vi "Initialize Ramp.vi"(7 "Sample Count":dbl, 8 "error in (no error)":errorcluster, 9 "End":dbl, 10 "Start":dbl, 11 "Ramp Stimulus in":refnum<class "Ramp Stimulus.lvclass">) -> (0 "error out":errorcluster, 3 "Ramp Stimulus out":refnum<class "Ramp Stimulus.lvclass">)   [LabVIEW 2015, in "Ramp Stimulus.lvclass"]
uses:
  Ramp Stimulus.lvclass
  Ramp Stimulus.lvclass/Ramp Stimulus.ctl
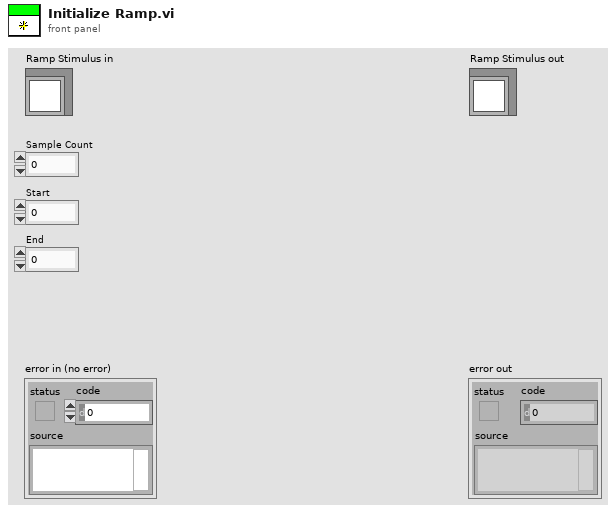
[diagram p1: front panel]
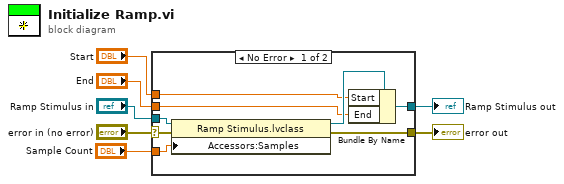
[diagram p0: block diagram]
diagram:
  n1 = case shown="No Error" "error in (no error)" {
    selector: "error in (no error)" -> [w13 w17]
    tunnel: [w12 w17] -> w6
    tunnel: [w8 w16] -> w4
    tunnel: "Ramp Stimulus in" -> [w15 w16]
    tunnel: "Start" -> [w11 _]
    tunnel: "End" -> [w10 _]
    tunnel: "Sample Count" -> [w9 _]
    frame No Error {
      n2 = property class="Ramp Stimulus.lvclass"(reference=w15, error in=w13, "Accessors:Samples"=w9) -> (reference out=w14:refnum<class "Ramp Stimulus.lvclass">, error out=w12:errorcluster)
      n3 = Bundle By Name(cluster=w14, "Start"=w11, "End"=w10) -> (w8:refnum<class "Ramp Stimulus.lvclass">)
    }
    frame Error {
    }
  }
  "error out" <- w6
  "Ramp Stimulus out" <- w4
